vi "TimePerTurnFGV.vi"(11 "Énum":enum16{"reset", "read", "home"}(ring)=enum."read") -> (2 "T1-T2 (ms)":u32, 3 "temps(s)/tour (360°)":dbl[](array[numeric]))   [LabVIEW 2020]
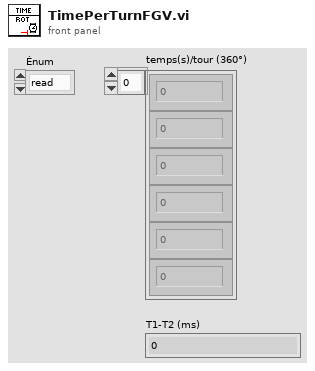
[diagram p1: front panel]
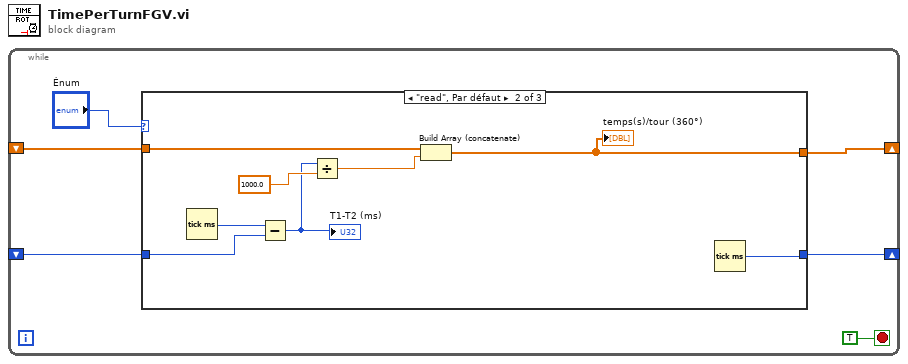
[diagram p0: block diagram]
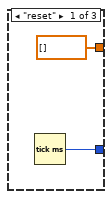
[diagram p2: hidden frame]
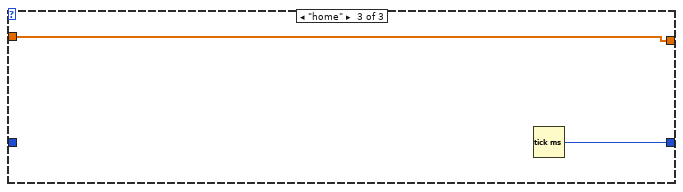
[diagram p3: hidden frame]
diagram:
  n1 = while {
    shift-right: [w4] -> _
    shift-left: _ -> [w1]
    shift-right: [w3] -> _
    shift-left: _ -> [w2]
    stop <- TRUE stop-if-true
    n2 = case shown="\"read\", Par défaut" "Énum" {
      tunnel: [dbl[] [] w10 w17] -> w4
      tunnel: [w7 w9 w18] -> w3
      tunnel: w2 -> [_ w15 _]
      tunnel: w1 -> [_ w11 w17]
      frame "reset" {
        n3 = Tick Count (ms)() -> (millisecond timer value=w7:u32)
      }
      frame "read", Default {
        n4 = Tick Count (ms)() -> (millisecond timer value=w16:u32)
        n5 = Subtract(x=w16, y=w15) -> (x-y=w13:u32)
        "T1-T2 (ms)" <- w13
        n6 = Divide(x=w13, y=1000.0) -> (x/y=w12:dbl)
        n7 = Build Array (concatenate)(w11, w12) -> (w10:dbl[])
        "temps(s)/tour (360°)" <- w10
        n8 = Tick Count (ms)() -> (millisecond timer value=w9:u32)
      }
      frame "home" {
        n9 = Tick Count (ms)() -> (millisecond timer value=w18:u32)
      }
    }
  }
